vi "Save Document.vi"(8 "error in (no error)":errorcluster, 11 "xwpfDocument in":refnum<class "xwpfDocument.lvclass">) -> (0 "error out":errorcluster, 3 "xwpfDocument out":refnum<class "xwpfDocument.lvclass">)   [LabVIEW 2017, in "Word_Specific.lvlib" / "xwpfDocument.lvclass"]
uses:
  xwpfDocument.lvclass
  xwpfDocument.lvclass/xwpfDocument.ctl
  C:/Program Files (x86)/National Instruments/LabVIEW 2017/vi.lib/BenjaminR/LabVIEW NPOI/lib/NPOI 2.1.1/NPOI.OOXML.dll
  Program Files (x86)/National Instruments/LabVIEW 2017/vi.lib/BenjaminR/LabVIEW NPOI/lib/NPOI 2.1.1/NPOI.OOXML.dll
  Support/File Stream/File Stream.lvlib
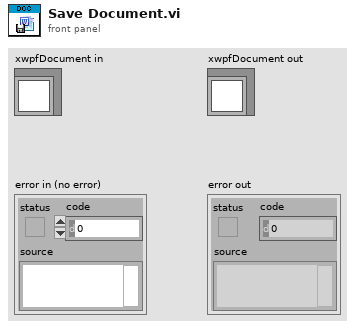
[diagram p1: front panel]
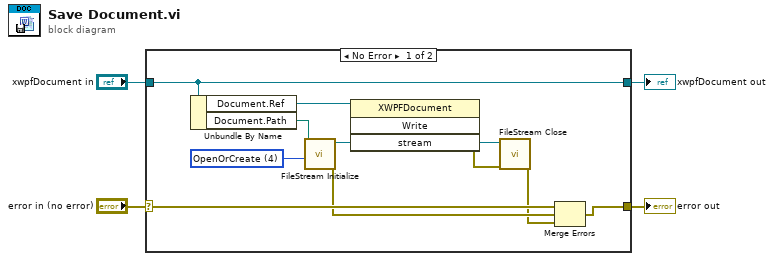
[diagram p0: block diagram]
diagram:
  n1 = case shown="No Error" "error in (no error)" {
    selector: "error in (no error)" -> [w14 w16]
    tunnel: [w7 w16] -> w3
    tunnel: [w13 w15] -> w1
    tunnel: "xwpfDocument in" -> [w13 w15]
    frame No Error {
      w10 = 4 items=["CreateNew"=1, "Create"=2, "Open"=3, "OpenOrCreate"=4, "Truncate"=5, "Append"=6] ("mode")
      n2 = Unbundle By Name(w13) -> ("Document.Ref"=w12:refnum<k24>, "Document.Path"=w11:path)
      n3 = call "FileStream Initialize.vi"("mode"=w10, "path"=w11) -> ("error out"=w6:errorcluster, "new reference"=w9:refnum<k24>)  [unwired: 8 in]
      n4 = invoke class="XWPFDocument" method="Write"(reference=w12, "stream"=w9) -> (error out=w8:errorcluster)  [unwired: 2 in, 3 out]
      n5 = call "FileStream Close.vi"("error in (no error)"=w8, "reference"=w9) -> ("error out"=w5:errorcluster)  [unwired: 9 in]
      n6 = Merge Errors(w14, w6, w5) -> (w7:errorcluster)
    }
    frame Error {
    }
  }
  "error out" <- w3
  "xwpfDocument out" <- w1
